vi "0x54_Cmd_prepare_table_parameter_(SubVI).vi"(10 "Parameters":T1 {"Номер колонки" min=0 step=4}, 11 "String in":string) -> (3 "String out":string)   [LabVIEW 2017, in "LV_Unicorn.lvlib"]
uses:
  LV_Unicorn.lvlib
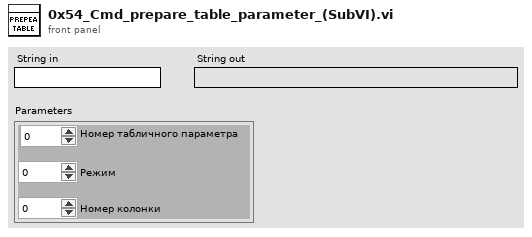
[diagram p1: front panel]
types:
  T1 = cluster{"Режим":i32, "Номер табличного параметра":i32, "Номер колонки":i32}
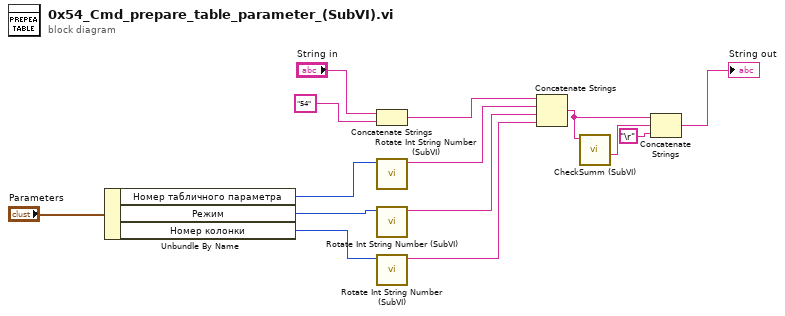
[diagram p0: block diagram]
diagram:
  n1 = Unbundle By Name("Parameters") -> ("Номер табличного параметра"=w4:i32, "Режим"=w3:i32, "Номер колонки"=w1:i32)
  n2 = Concatenate Strings("String in", "54" ("string")) -> (w12:string)
  n3 = call "Rotate Int String Number (SubVI).vi"("Int Number In"=w4) -> ("Orig String"=w6:string)  [unwired: 8 in, 2 out]
  n4 = call "Rotate Int String Number (SubVI).vi"("Int Number In"=w3) -> ("Orig String"=w7:string)  [unwired: 8 in, 2 out]
  n5 = call "Rotate Int String Number (SubVI).vi"("Int Number In"=w1) -> ("Orig String"=w5:string)  [unwired: 8 in, 2 out]
  n6 = Concatenate Strings(w12, w6, w7, w5) -> (w9:string)
  n7 = call "CheckSumm (SubVI).vi"("Input String"=w9) -> ("CheckSumm"=w8:string)  [unwired: 7 in, 3 out]
  n8 = Concatenate Strings(w9, w8, "\r") -> (→"String out":string)
